vi "data summary to string.vi"(1 "data summary":T1) -> (0 "data summary string":string)   [LabVIEW 2016]
uses:
  Type Def Ctrls/RT ctrls/data summary.ctl
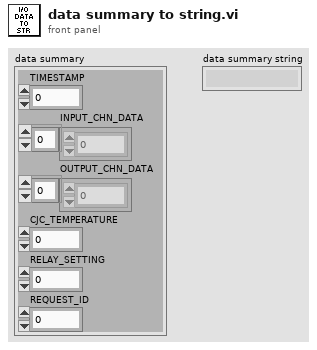
[diagram p1: front panel]
types:
  T1 = typedef "data summary.ctl" = cluster{"TIMESTAMP":dbl, "INPUT_CHN_DATA":sgl[], "OUTPUT_CHN_DATA":sgl[], "CJC_TEMPERATURE":sgl, "RELAY_SETTING":u32, "REQUEST_ID":u64}
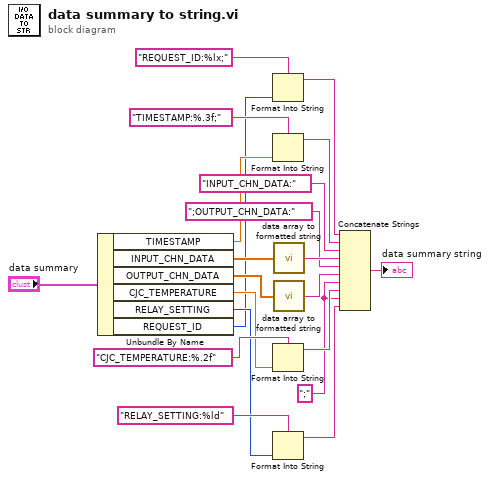
[diagram p0: block diagram]
diagram:
  w12 = ";" ("string")
  n1 = Unbundle By Name("data summary") -> ("TIMESTAMP"=w8:dbl, "INPUT_CHN_DATA"=w7:sgl[], "OUTPUT_CHN_DATA"=w6:sgl[], "CJC_TEMPERATURE"=w5:sgl, "RELAY_SETTING"=w4:u32, "REQUEST_ID"=w2:u64)
  n2 = Format Into String(format string="REQUEST_ID:%lx;", w2) -> (resulting string=w1:string)  [unwired: 2 in, 1 out]
  n3 = Format Into String(format string="TIMESTAMP:%.3f;", w8) -> (resulting string=w18:string)  [unwired: 2 in, 1 out]
  n4 = Format Into String(format string="CJC_TEMPERATURE:%.2f", w5) -> (resulting string=w13:string)  [unwired: 2 in, 1 out]
  n5 = Format Into String(format string="RELAY_SETTING:%ld", w4) -> (resulting string=w11:string)  [unwired: 2 in, 1 out]
  n6 = call "data array to formatted string.vi"("data array"=w7) -> ("formatted string"=w17:string)
  n7 = call "data array to formatted string.vi"("data array"=w6) -> ("formatted string"=w14:string)
  n8 = Concatenate Strings(w1, w18, "INPUT_CHN_DATA:" ("string"), w17, ";OUTPUT_CHN_DATA:" ("string"), w14, w12, w13, w12, w11) -> (→"data summary string":string)
